vi "Actor.vi"(5 "Queue of Error":refnum<queue>, 7 "Queue of Self":refnum<queue>, 8 "Self Alias":string, 9 "Caller":refnum<data-value>, 10 "Caller Alias":string, 11 "Actor":refnum<class "Actor.lvclass">) -> ()   [LabVIEW 2021, in "jettl.lvlib" / "jettl Queue Actor.lvlib" / "jettl Queue Actor.lvclass"]
uses:
  jettl Queue Actor.lvclass
  Actor/Msg/Msg.lvclass
  Actor/Actor/Actor.lvclass
  C:/git/jettl/src/Actor/Actor/Actor.lvclass
  State/Nominal State/Nominal State.lvclass
  C:/git/jettl/src/jettl/jettl Queue Actor/State/State/State.lvclass
  Actor/Queue Actor/Queue Actor.lvclass
  jettl Queue Actor.lvclass/jettl Queue Actor.ctl
  jettl.lvlib
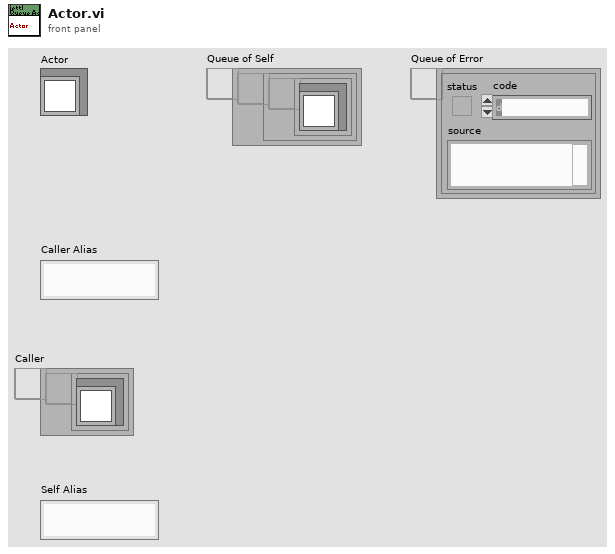
[diagram p1: front panel]
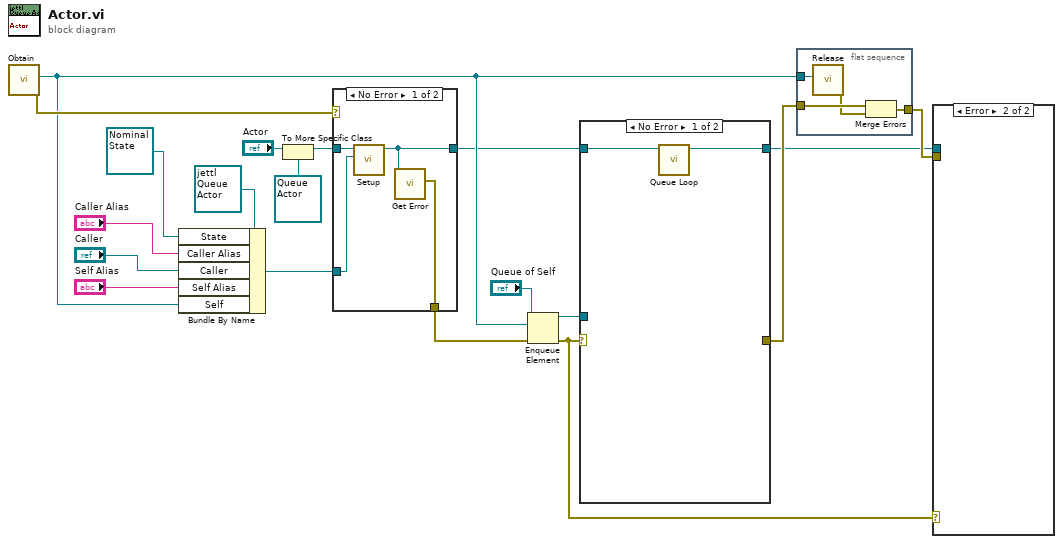
[diagram p0: block diagram]
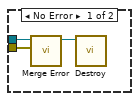
[diagram p2: hidden frame]
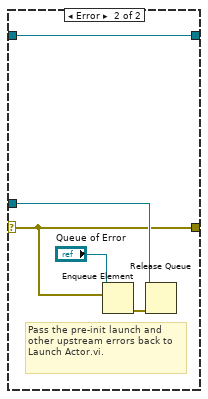
[diagram p4: hidden frame]
diagram:
  n1 = call "Obtain.vi"() -> ("error out"=w16:errorcluster, "Queue"=w2:refnum<data-value>)  [unwired: 10 in]
  n2 = Bundle By Name(cluster=refnum<class "jettl Queue Actor.lvclass"> refnum ("Self Actor in"), "State"=refnum<class "Nominal State.lvclass"> refnum ("LVCAM.lvlib:Msging Self Actor State.lvclass"), "Caller Alias"="Caller Alias", "Caller"="Caller", "Self Alias"="Self Alias", "Self"=w2) -> (w8:refnum<class "jettl Queue Actor.lvclass">)
  n3 = To More Specific Class(target class=refnum<class "Queue Actor.lvclass"> refnum ("Queue Actor.lvclass"), reference="Actor") -> (specific class reference=w4:refnum<class "Queue Actor.lvclass">)  [unwired: 1 in, 1 out]
  n4 = case shown="No Error" w16 {
    selector: w16 -> [_ w25]
    tunnel: w4 -> [w23 w24]
    tunnel: [w22 w24] -> w1
    tunnel: [w21 w25] -> w18
    tunnel: w8 -> [w20 _]
    frame No Error {
      n5 = call-dynamic "Setup.vi"("Actor"=w20, "Actor in"=w23) -> ("Actor out"=w22:refnum<class "Queue Actor.lvclass">)  [unwired: 9 in]
      n6 = call-dynamic "Get Error.vi"("Actor in"=w22) -> ("Error"=w21:errorcluster)  [unwired: 10 in]
    }
    frame Error {
    }
  }
  n7 = Enqueue Element(queue="Queue of Self", element=w2, error in (no error)=w18) -> (queue out=w19:refnum<queue>, error out=w17:errorcluster)  [unwired: 1 in, 1 out]
  n8 = case shown="No Error" w17 {
    selector: w17 -> [_ w29]
    tunnel: w1 -> [w27 w32]
    tunnel: [_ w29] -> w15
    tunnel: [w26 w32] -> w6
    tunnel: w19 -> [_ w31]
    frame No Error {
      n9 = call "Queue Loop.vi"("Queue Actor in"=w27) -> ("Queue Actor out"=w26:refnum<class "Queue Actor.lvclass">)  [unwired: 10 in]
    }
    frame Error {
      # "Pass the pre-init launch and other upstream errors back to Launch Actor.vi."
      n10 = Enqueue Element(queue="Queue of Error", element=w29) -> (error out=w30:errorcluster)  [unwired: 2 in, 2 out]
      n11 = Release Queue(queue=w31, error in (no error)=w30) -> ()  [unwired: 1 in, 3 out]
    }
  }
  n12 = flat-sequence {
    tunnel: w15 -> [w35]
    tunnel: w2 -> [w36]
    tunnel: [w33] -> w14
    frame #0 {
      n13 = call "Release.vi"("Queue"=w36) -> ("error out"=w34:errorcluster)  [unwired: 10 in]
      n14 = Merge Errors(w35, w34) -> (w33:errorcluster)
    }
  }
  n15 = case shown="Error" w17 {
    tunnel: w14 -> [w37 _]
    tunnel: w6 -> [w39 _]
    frame No Error {
      n16 = call-dynamic "Merge Error.vi"("Error"=w37, "Set Error in"=w39) -> ("Set Error out"=w38:refnum<class "Queue Actor.lvclass">)  [unwired: 9 in]
      n17 = call-dynamic "Destroy.vi"("Actor in"=w38) -> ()  [unwired: 11 in]
    }
    frame Error {
    }
  }
